vi "Bp_monitor_hack.vi"() -> ()   [LabVIEW 2020]
uses:
  <vilib>/Analysis/baseanly.llb/Mean (DBL).vi
  <vilib>/Analysis/NI_AALBase.lvlib
panel:
  out "Measured Cuff Pressure [mmHG] =":dbl format="%.2f"
  out "Setpoint Cuff Pressure [mmHg] =":dbl caption="Hold the Cuff Pressure [mmHg]" format="%#g"
  in  "Omron Ready":bool caption="E1 Displayed ?"
  out "Pressure Exceeded":bool
  out "AC Cuff Pressure":dynamicdata(graph)
  out "DC Cuff Pressure [mmHg]":dynamicdata(graph)
  in  "Stop Expt":bool caption="Stop Experiment"
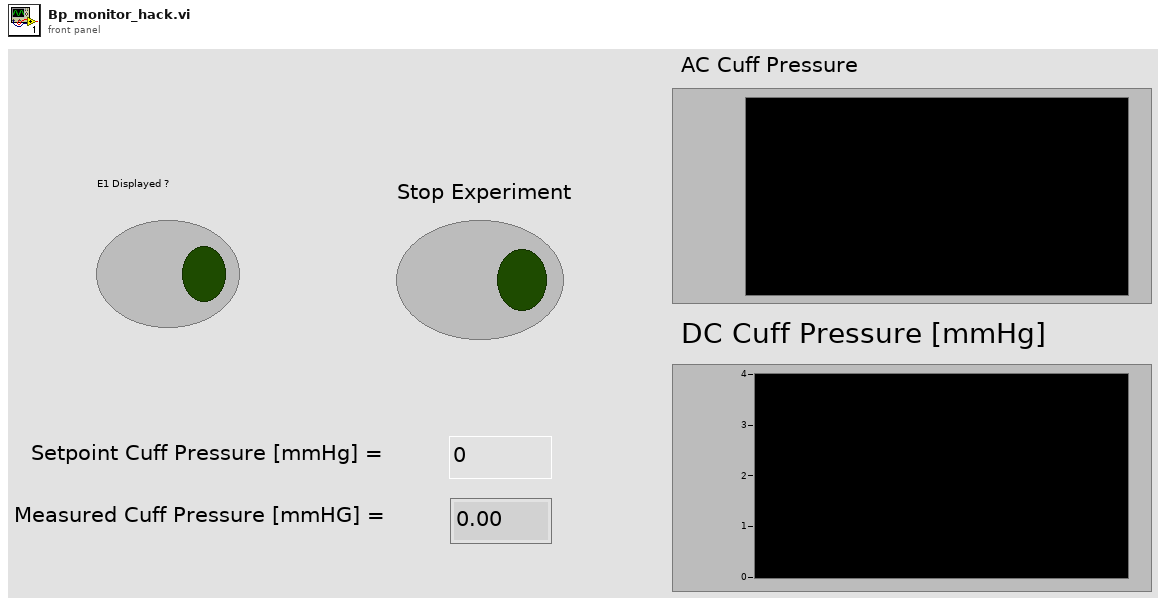
[diagram p1: front panel]
types:
  T1 = enum16{"Increase Pressure", "Reduce Pressure", "Hold Pressure", "Zero State (Omron)"}
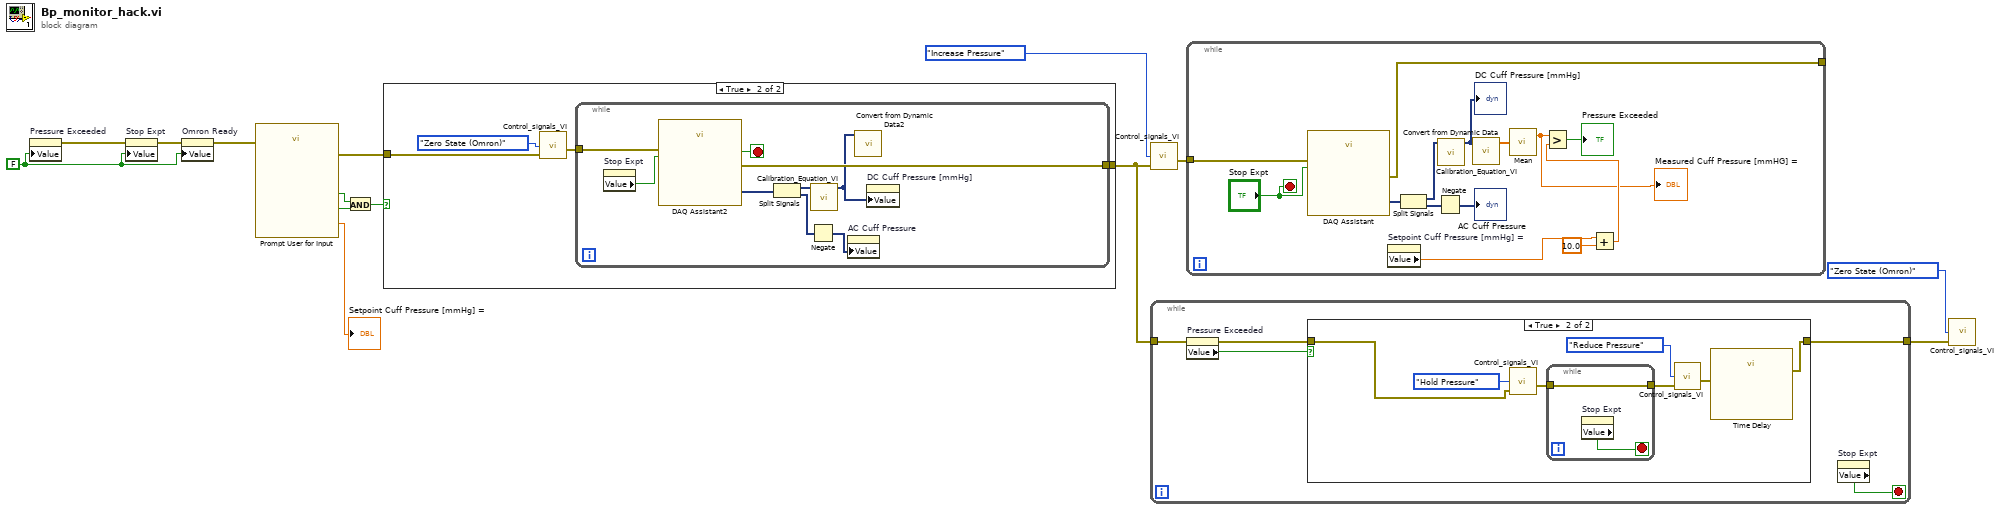
[diagram p0: block diagram]
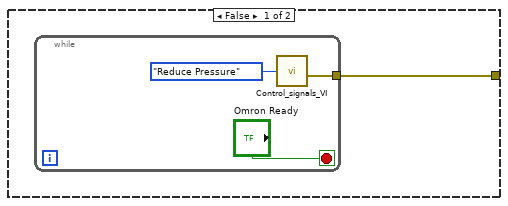
[diagram p2: hidden frame]
diagram:
  w10 = FALSE ("Stop Holding Pressure")
  n1 = property on="Pressure Exceeded" class="Bool (strict)"("Value"=w10) -> (error out=w8:errorcluster)  [unwired: 2 in, 1 out]
  n2 = property on="Stop Expt" class="Bool (strict)"(error in=w8, "Value"=w10) -> (error out=w13:errorcluster)  [unwired: 1 in, 1 out]
  n3 = property on="Omron Ready" class="Bool (strict)"(error in=w13, "Value"=w10) -> (error out=w7:errorcluster)  [unwired: 1 in, 1 out]
  n4 = call "Prompt User for Input"("error in (no error)"=w7) -> ("Hold the Cuff Pressure [mmHg]"=→"Setpoint Cuff Pressure [mmHg] =":dbl, "Record Omron Data"=w5:bool, "OK"=w6:bool, "error out"=w3:errorcluster)  [unwired: 15 in]
  n5 = And(x=w6, y=w5) -> (x .and. y?=w4:bool)
  n6 = case shown="True" w4 {
    tunnel: w3 -> [_ w21]
    tunnel: [w15 w20] -> w2
    frame False {
      n7 = while {
        tunnel: [w17] -> w15
        stop <- "Omron Ready" stop-if-true
        n8 = call "Control_signals_VI.vi"("Input"=T1."Reduce Pressure") -> ("error out"=w17:errorcluster)  [unwired: 5 in, 1 out]
      }
    }
    frame True {
      n9 = call "Control_signals_VI.vi"("Input"=T1."Zero State (Omron)", "error in"=w21) -> ("error out"=w19:errorcluster)  [unwired: 4 in, 1 out]
      n10 = while {
        tunnel: [w26] -> w20
        tunnel: w19 -> [w25]
        stop <- w27 stop-if-true
        n11 = property on="Stop Expt" class="Bool (strict)"() -> ("Value"=w24:bool)  [unwired: 2 in, 2 out]
        n12 = call "DAQ Assistant2"("error in"=w25, "stop (F)"=w24) -> ("data"=w29:dynamicdata, "stopped"=w27:bool, "error out"=w26:errorcluster)  [unwired: 14 in, 1 out]
        n13 = Split Signals(w29) -> (w31:dynamicdata, w30:dynamicdata)  [unwired: 2 in]
        n14 = Negate(x=w30) -> (-x=w28:dynamicdata)
        n15 = call "Calibration_Equation_VI.vi"("Dynamic Data in"=w31) -> ("Dynamic Data out"=w23:dynamicdata)  [unwired: 10 in]
        n16 = property on="AC Cuff Pressure" class="WFChart (strict)"("Value"=w28) -> ()  [unwired: 2 in, 2 out]
        n17 = call "Convert from Dynamic Data2"("Dynamic Data Type"=w23) -> ()  [unwired: 3 in, 1 out]
        n18 = property on="DC Cuff Pressure [mmHg]" class="WFChart (strict)"("Value"=w23) -> ()  [unwired: 2 in, 2 out]
      }
    }
  }
  n19 = call "Control_signals_VI.vi"("Input"=T1."Increase Pressure", "error in"=w2) -> ("error out"=w11:errorcluster)  [unwired: 4 in, 1 out]
  n20 = while {
    tunnel: w2 -> [w35]
    tunnel: [w33] -> w9
    stop <- w32 stop-if-true
    n21 = property on="Pressure Exceeded" class="Bool (strict)"(error in=w35) -> (error out=w34:errorcluster, "Value"=w36:bool)  [unwired: 1 in, 1 out]
    n22 = case shown="True" w36 {
      tunnel: w34 -> [w37 w38]
      tunnel: [w37 w39] -> w33
      frame False {
      }
      frame True {
        n23 = call "Control_signals_VI.vi"("Input"=T1."Hold Pressure", "error in"=w38) -> ("error out"=w43:errorcluster)  [unwired: 4 in, 1 out]
        n24 = while {
          tunnel: w43 -> [w46]
          tunnel: [w46] -> w41
          stop <- w45 stop-if-true
          n25 = property on="Stop Expt" class="Bool (strict)"() -> ("Value"=w45:bool)  [unwired: 2 in, 2 out]
        }
        n26 = call "Control_signals_VI.vi"("Input"=T1."Reduce Pressure", "error in"=w41) -> ("error out"=w40:errorcluster)  [unwired: 4 in, 1 out]
        n27 = call "Time Delay"("error in (no error)"=w40) -> ("error out"=w39:errorcluster)  [unwired: 10 in]
      }
    }
    n28 = property on="Stop Expt" class="Bool (strict)"() -> ("Value"=w32:bool)  [unwired: 2 in, 2 out]
  }
  n29 = while {
    tunnel: [w54] -> _
    tunnel: w11 -> [w59]
    stop <- "Stop Expt" stop-if-true
    n30 = call "DAQ Assistant"("error in"=w59, "stop (T)"="Stop Expt") -> ("data"=w60:dynamicdata, "error out"=w54:errorcluster)  [unwired: 15 in, 1 out]
    n31 = property on="Setpoint Cuff Pressure [mmHg] =" class="DigNum (strict)"() -> ("Value"=w50:dbl)  [unwired: 2 in, 2 out]
    n32 = Split Signals(w60) -> (w58:dynamicdata, w53:dynamicdata)  [unwired: 2 in]
    n33 = Negate(x=w53) -> (-x=→"AC Cuff Pressure":dynamicdata)
    n34 = call "Calibration_Equation_VI.vi"("Dynamic Data in"=w58) -> ("Dynamic Data out"=w57:dynamicdata)  [unwired: 10 in]
    "DC Cuff Pressure [mmHg]" <- w57
    n35 = call "Convert from Dynamic Data"("Dynamic Data Type"=w57) -> ("Array"=w56:dbl[])  [unwired: 3 in]
    n36 = call-poly <vilib>:"Mean.vi"("X"=w56) -> ("mean"=w47:dbl)  [unwired: 1 out]
    "Measured Cuff Pressure [mmHG] =" <- w47
    n37 = Add(x=w50, y=10.0) -> (x+y=w48:dbl)
    n38 = Greater?(x=w47, y=w48) -> (0:→"Pressure Exceeded":bool)
  }
  n39 = call "Control_signals_VI.vi"("Input"=T1."Zero State (Omron)", "error in"=w9) -> ()  [unwired: 4 in, 2 out]
